vi "Config List Sweep.vi"(0 "VISA Resource Name":refnum<visa-resource-name>, 1 "List Define (0:User Defined)":u16(ring) items=["User Defined", "Preset Default", "Load from Step"], 5 "Frequency (1003.0)":dbl[](array[numeric]) format="%.2f", 7 "Power (-135.00)":dbl[](array[numeric]) format="%.2f", 9 "Dwell (2.00)":dbl[](array[numeric]) format="%.2f", 11 "error in (no error)":errorcluster {"code" format="%.0x"}) -> (4 "VISA Resource Name Out":refnum<visa-resource-name>, 15 "error out":errorcluster {"code" format="%.0x"})   [LabVIEW 2012, in "Agilent ESG Series.lvlib"]
doc: "This VI is used to set the controls and the parameters associated with frequency and/or power step sweep."
uses:
  <instrlib>/Agilent ESG Series/Agilent ESG Series.lvlib
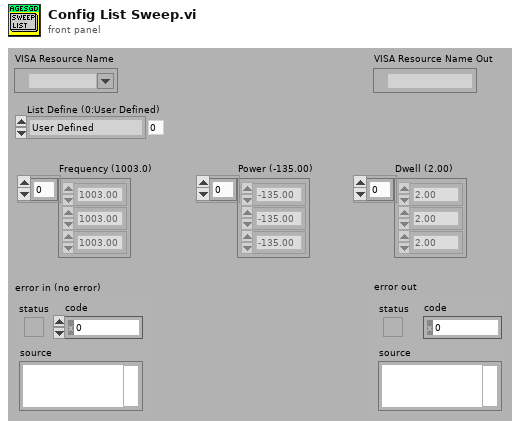
[diagram p1: front panel]
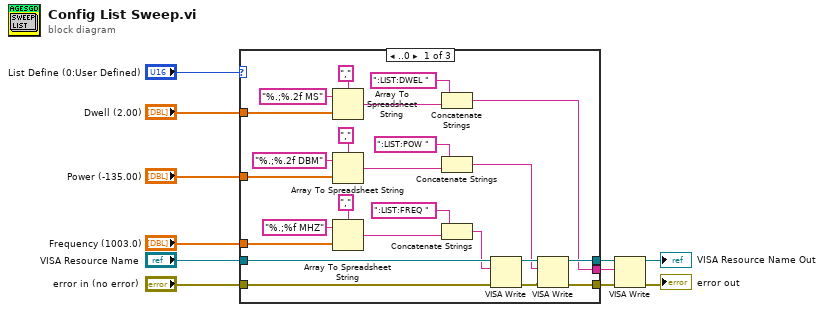
[diagram p0: block diagram]
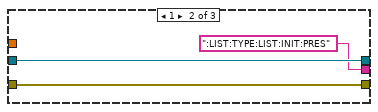
[diagram p2: hidden frame]
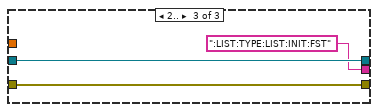
[diagram p3: hidden frame]
diagram:
  n1 = case shown="..0" "List Define (0:User Defined)" {
    tunnel: [w14 ":LIST:TYPE:LIST:INIT:PRES" ":LIST:TYPE:LIST:INIT:FST"] -> w5
    tunnel: [w35 w37 w40] -> w8
    tunnel: [w33 w38 w41] -> w9
    tunnel: "Dwell (2.00)" -> [w19 _ _]
    tunnel: "Power (-135.00)" -> [w18 _ _]
    tunnel: "Frequency (1003.0)" -> [w17 _ _]
    tunnel: "error in (no error)" -> [w16 w37 w40]
    tunnel: "VISA Resource Name" -> [w15 w38 w41]
    frame ..0 {
      n2 = Array To Spreadsheet String(delimiter (Tab)=",", array=w19, 3:"%.;%.2f MS" ("format string")) -> (spreadsheet string=w25:string)
      n3 = Array To Spreadsheet String(delimiter (Tab)=",", array=w18, 3:"%.;%.2f DBM" ("format string")) -> (spreadsheet string=w26:string)
      n4 = Array To Spreadsheet String(delimiter (Tab)=",", array=w17, 3:"%.;%f MHZ" ("format string")) -> (spreadsheet string=w23:string)
      n5 = Concatenate Strings(":LIST:DWEL ", w25) -> (w14:string)
      n6 = Concatenate Strings(":LIST:POW ", w26) -> (w12:string)
      n7 = Concatenate Strings(":LIST:FREQ ", w23) -> (w13:string)
      n8 = VISA Write(VISA resource name=w15, write buffer=w13, error in (no error)=w16) -> (VISA resource name out=w32:refnum<visa-resource-name>, error out=w34:errorcluster)  [unwired: 1 out]
      n9 = VISA Write(VISA resource name=w32, write buffer=w12, error in (no error)=w34) -> (VISA resource name out=w33:refnum<visa-resource-name>, error out=w35:errorcluster)  [unwired: 1 out]
    }
    frame 1 {
    }
    frame 2.. {
    }
  }
  n10 = VISA Write(VISA resource name=w9, write buffer=w5, error in (no error)=w8) -> (VISA resource name out=→"VISA Resource Name Out":refnum<visa-resource-name>, error out=→"error out":errorcluster)  [unwired: 1 out]
